vi "5785_p2p_IQ_gen_1_6GHz_max_and_pulse_detector.vi"() -> ()   [LabVIEW 2021]
uses:
  pulse detector/FPGA/reciver params.ctl
  <vilib>/Platform/TimedLoop/XDataNode/timing_clust.ctl
  <vilib>/Platform/TimedLoop/XDataNode/nitl_modes.ctl
  <vilib>/Platform/TimedLoop/XDataNode/wakeup.ctl
  <vilib>/rvi/Emulation/niFpgaSctlEmulationGetInTimedLoop.vi
  <vilib>/rvi/Emulation/niFpgaEmulationReportErrorSimple.vi
  <vilib>/rvi/Emulation/niFpgaGetClockAttributes.vi
  <vilib>/rvi/Emulation/niFpgaCriticalErrorInLSC.vi
  <instrlib>/_niInstr/Basic Elements/v1/FPGA/Private/Count Up U64.vi
  <vilib>/rvi/interface/RandomDataEmulation/nirviRandomDataMultiElementFPGAFIFO.vi
  <instcachedir>/0/nirviRandomDataMultiElementFPGAFIFO_3E9965BA1FAD4E7B8DABA31768A09B1F.lvgen/nirviRandomDataMultiElementFPGAFIFO_3E9965BA1FAD4E7B8DABA31768A09B1F_000.vi
  <vilib>/rvi/interface/RandomDataEmulation/niFpgaRandomDataHandleErrors.vi
  <instrlib>/_niInstr/Basic Elements/v1/FPGA/Private/Count Up U32.vi
  <vilib>/Platform/TimedLoop/XDataNode/XDataNode.xnode
  <vilib>/rvi/DataTransferAndStorage/Container/XNode/niFpgaContainer.xnode
  <vilib>/rvi/FIFO/Fifo_Resource/nirvififoEmulationP2P.vi
  <vilib>/rvi/interface/RandomDataEmulation/nirviRandomDataFpgaMultiElementTemplate.vi
  <vilib>/Platform/TimedLoop/XDataNode/XDNodeRunTimeDep.lvlib
  <instrlib>/_niInstr/Basic Elements/v1/FPGA/niInstr Basic Elements v1 FPGA.lvlib
panel:
  out "fft_output":u64
  out "last pdw":u64[](array[numeric])
  out "raw IQ":u32
  in  "reciver_params 2":T1
  out "lost sampels":u32
  in  "P2P empty room for runing":u32=2000
  out "pulse TX status":T2
  in  "reset system clock":bool
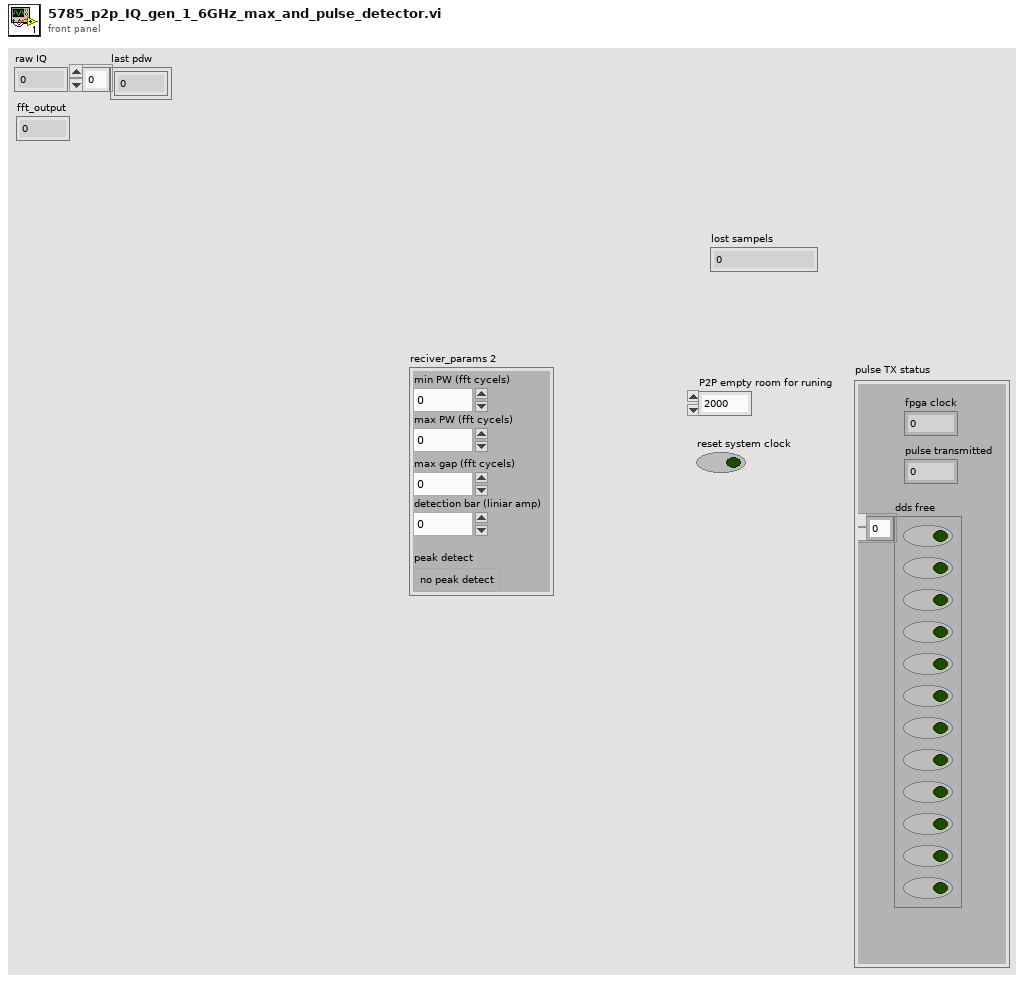
[diagram p1: front panel]
types:
  T1 = typedef "reciver params.ctl" = cluster{"min PW (fft cycels)":u16, "max PW (fft cycels)":u16, "max gap (fft cycels)":u8, "detection bar (liniar amp)":fxp<+,64,63>, "peak detect":bool}
  T2 = cluster{"fpga clock":u64, "pulse transmitted":u32, "dds free":bool[]}
  T3 = typedef "XDNodeRunTimeDep.lvlib/timing_clust.ctl" = cluster{"Expected End [f-1]":u64, "Actual End [f-1]":u64, "Finished Late? [f-1]":bool, "Expected End [i-1]":u64, "Actual End [i-1]":u64, "Finished Late? [i-1]":bool, "Expected Start [i]":u64, "Actual Start [i]":u64, "Expected Start [f]":u64, "Actual Start [f]":u64, "Source Name":string, "Structure Name":string, "Period":i64, "Deadline":i64, "Offset":i64, "Start":i64, "Priority":i32, "Timeout":i32, "Mode":T4, "Wakeup Reason":T5, "Error":errorcluster, "Source Type":string, "Secondary Source Type":string, "Global End Time":u64, "Global Start Time":u64, "Frame Duration":u64, "Iteration Duration":u64, "Assigned CPU":i32, "I/O Scan Engine Mode":u32}
  T4 = typedef "XDNodeRunTimeDep.lvlib/nitl_modes.ctl" = enum32{"No Change", "Process missed periods, maintain original phase", "Discard missed periods, maintain original phase", "Process missed periods, ignore original phase", "Discard missed periods, ignore original phase"}
  T5 = typedef "XDNodeRunTimeDep.lvlib/wakeup.ctl" = enum32{"Normal", "Aborted", "Asynchronous wakeup", "Timing source error", "Timed loop error", "Timeout"}
  T6 = typedef "niInstr DSP v1 Shared.lvlib/IQ Data.ctl" = cluster{"I":fxp<+/-,18,1>, "Q":fxp<+/-,18,1>, "overflow":bool}
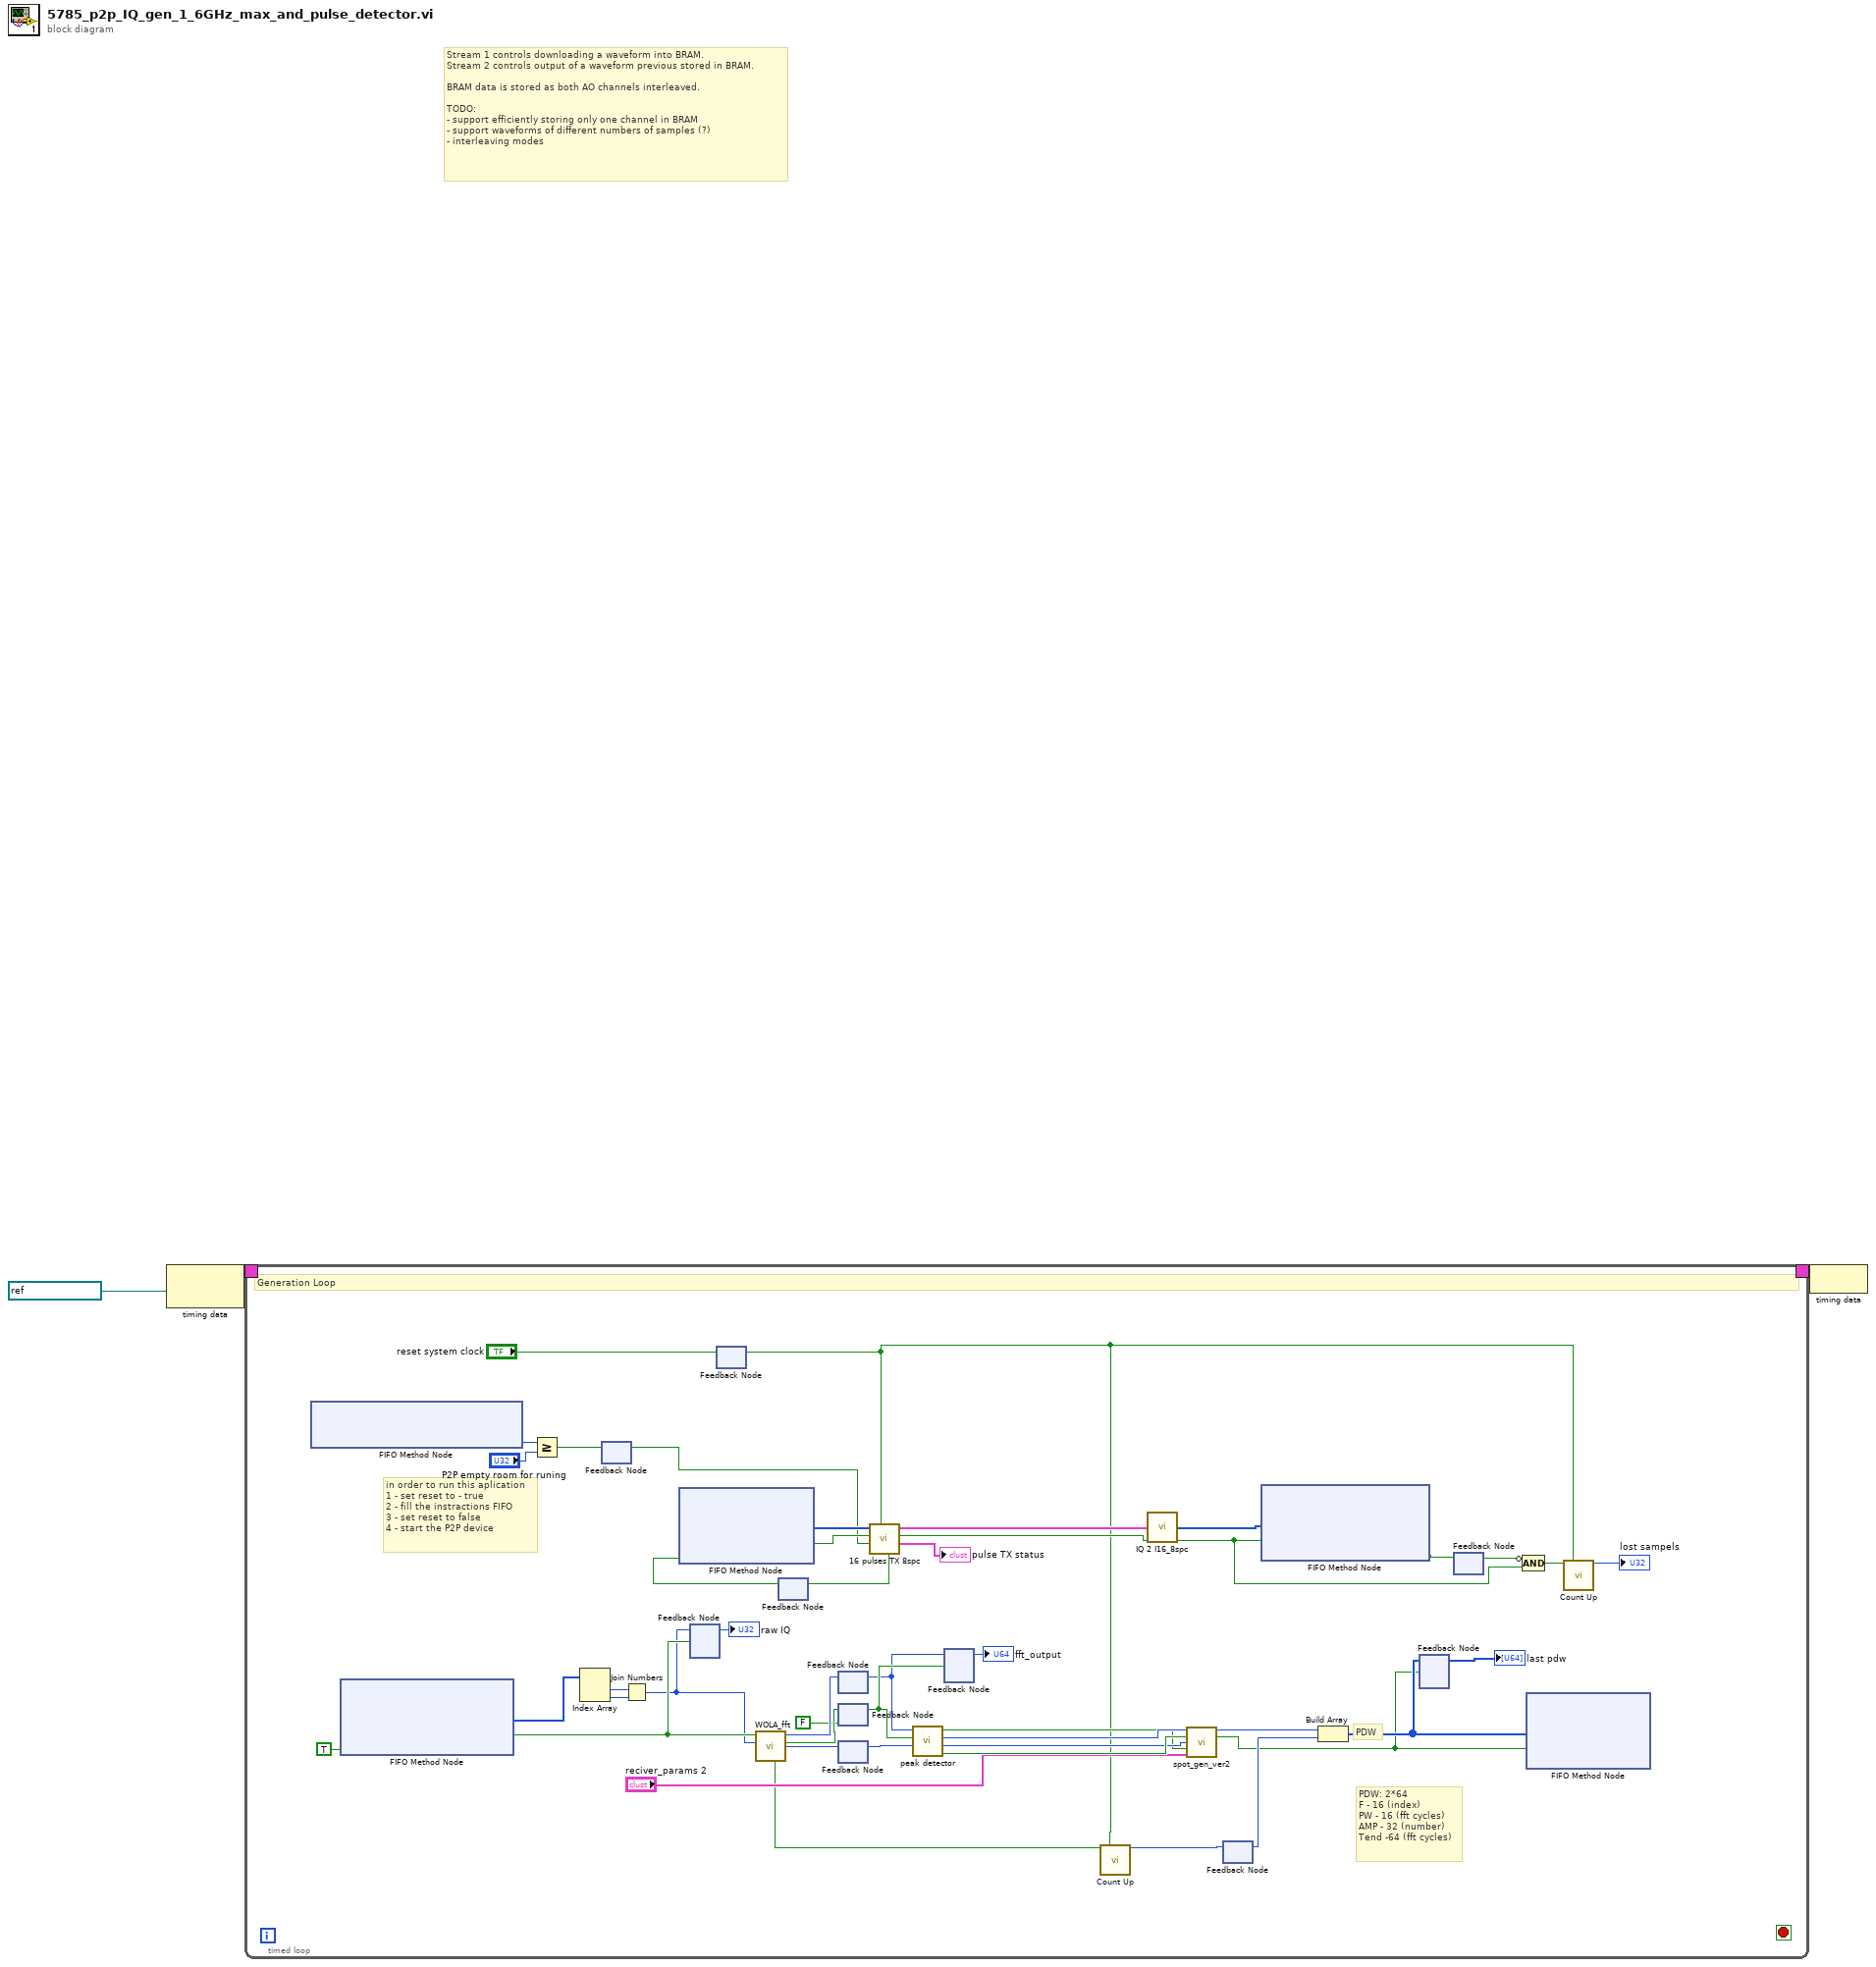
[diagram p0: block diagram]
diagram:
  # "Stream 1 controls downloading a waveform into BRAM.\nStream 2 controls output of a waveform previous stored in BRAM.\n\nBRAM data is stored as both AO channels interleaved.\n\nTODO:\n- support efficiently storing only one channel in BRAM\n- support waveforms of different numbers of samples (?)\n- interleaving modes"
  n1 = node-c288(refnum<k21> "PXIe_CLK200" ("Source Name")) -> (w3:T3)
  n2 = timed-loop {
    timing: w3 -> [_]
    timing-out: [_] -> w2
    stop <- _ stop-if-true
    # "PDW: 2*64\nF - 16 (index)\nPW - 16 (fft cycles)\nAMP - 32 (number)\nTend -64 (fft cycles)"
    # "PDW"
    # "in order to run this aplication\n1 - set reset to - true\n2 - fill the instractions FIFO\n3 - set reset to false\n4 - start the P2P device"
    # "Generation Loop"
    n3 = xnode ("FIFO Method Node")() -> ("Number of Elements to Write"=w34:u32)  [unwired: 1 in, 1 out]
    n4 = xnode ("FIFO Method Node")("Ready for Output"=TRUE) -> ("Element"=w16:i16[], "Output Valid"=w12:bool)  [unwired: 1 in, 1 out]
    n5 = Greater Or Equal?(x=w34, y="P2P empty room for runing") -> (x >= y?=w42:bool)
    n6 = Index Array(array=w16) -> (element #1=w14:i16, element #2=w15:i16)  [unwired: 2 in]
    n7 = feedback #1() -> (w43:bool)  [unwired: 1 in]
    n8 = feedback-in #1(w42) -> ()
    n9 = Join Numbers(hi=w14, lo=w15) -> ((hi.lo)=w11:u32)
    n10 = feedback #2() -> (→"raw IQ":u32)  [unwired: 1 in]
    n11 = feedback-in #2(w11, w12) -> ()
    n12 = feedback-in #3("reset system clock") -> ()
    n13 = feedback #3() -> (w17:bool)  [unwired: 1 in]
    n14 = call "WOLA_fft.vi"("data in"=w11, "input valid"=w12) -> ("data index"=w26:u16, "output valid"=w28:bool, "fft_output"=w29:u64, "new fft cycle"=w19:bool)  [unwired: 6 in]
    n15 = feedback #4() -> (w47:bool)  [unwired: 1 in]
    n16 = xnode ("FIFO Method Node")("Ready for Output"=w47) -> ("Element"=w46:u64[], "Output Valid"=w45:bool)  [unwired: 1 in, 1 out]
    n17 = feedback #5() -> (w5:u64)  [unwired: 1 in]
    n18 = feedback-in #5(w29) -> ()
    n19 = feedback #6(FALSE ("output valid 2")) -> (w6:bool)
    n20 = feedback-in #6(w28) -> ()
    n21 = feedback #7() -> (w25:u16)  [unwired: 1 in]
    n22 = feedback-in #7(w26) -> ()
    n23 = call "16 pulses TX 8spc.vi"("reset system clock"=w17, "IQ_run"=w43, "PDW input Valid"=w45, "array PDW"=w46) -> ("pulse TX status"=→"pulse TX status":T2, "output valid"=w32:bool, "IQ out"=w33:T6[], "ready for input"=w48:bool)  [unwired: 4 in]
    n24 = feedback-in #4(w48) -> ()
    n25 = call "peak detector.vi"("data index"=w25, "output valid in"=w6, "fft_output"=w5) -> ("output valid"=w23:bool, "adress"=w22:u16, "amplitude"=w24:u32, "peak"=w21:bool)  [unwired: 5 in]
    n26 = feedback #8() -> (→"fft_output":u64)  [unwired: 1 in]
    n27 = feedback-in #8(w5, w6) -> ()
    n28 = call-poly <instrlib>:"Count Up.vi"("increment"=w19, "reset"=w17) -> ("count out"=w18:u64)  [unwired: 13 in]
    n29 = call "IQ 2 I16_8spc.vi"("IQ in"=w33) -> ("interleaved IQ array"=w36:i16[])
    n30 = call "spot_gen_ver2.vi"("amp"=w24, "input valid"=w23, "data index"=w22, "peak"=w21, "reciver_params"="reciver_params 2") -> ("PDW"=w31:u64, "output valid"=w8:bool)  [unwired: 8 in, 1 out]
    n31 = feedback #9() -> (w30:u64)  [unwired: 1 in]
    n32 = feedback-in #9(w18) -> ()
    n33 = xnode ("FIFO Method Node")("Element"=w36, "Input Valid"=w32) -> ("Ready for Input"=w35:bool)  [unwired: 1 in, 1 out]
    n34 = Build Array(w31, w30) -> (w9:u64[])
    n35 = feedback #10() -> (→"last pdw":u64[])  [unwired: 1 in]
    n36 = feedback-in #10(w9, w8) -> ()
    n37 = feedback-in #11(w35) -> ()
    n38 = feedback #11() -> (w40:bool)  [unwired: 1 in]
    n39 = Compound Arithmetic op=AND(invert w40, w32) -> (w39:bool)
    n40 = xnode ("FIFO Method Node")("Element"=w9, "Input Valid"=w8) -> ()  [unwired: 1 in, 2 out]
    n41 = call-poly <instrlib>:"Count Up.vi"("increment"=w39, "reset"=w17) -> ("count out"=→"lost sampels":u32)  [unwired: 13 in]
  }
  n42 = node-c288(w2) -> ()
